vi "generate_CSV.vi"(11 "Array":string[](array[string])) -> (4 "error out":errorcluster)   [LabVIEW 2020, in "FBN_LATM.lvlib"]
uses:
  FBN_LATM.lvlib
  <vilib>/Utility/file.llb/Write Delimited Spreadsheet (string).vi
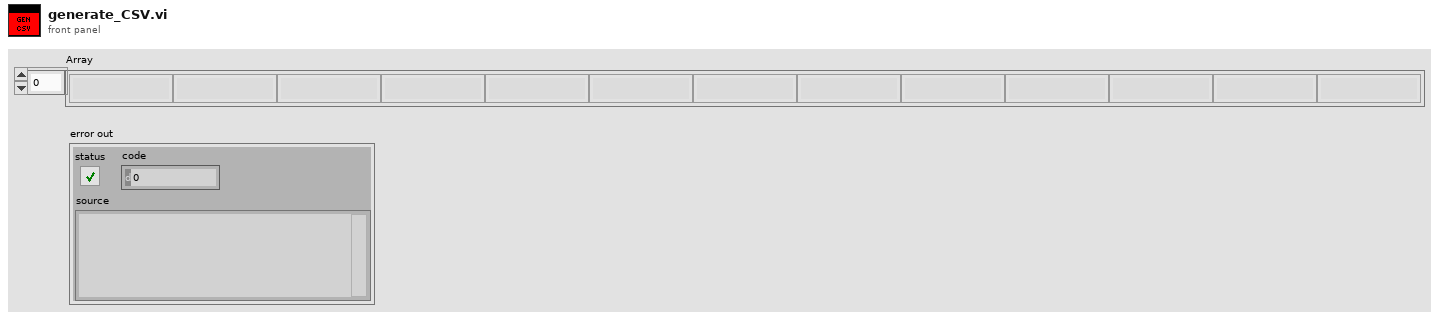
[diagram p1: front panel]
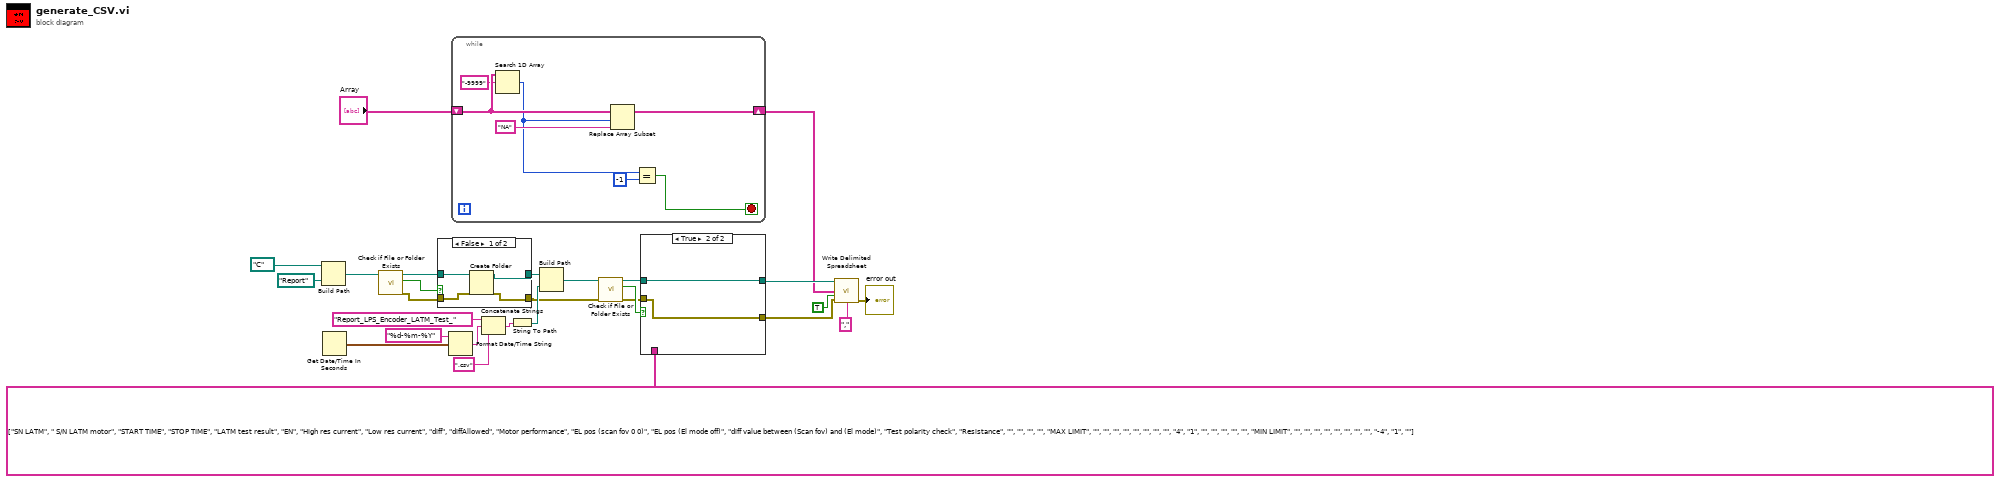
[diagram p0: block diagram]
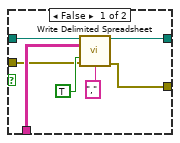
[diagram p2: hidden frame]
diagram:
  n1 = Build Path(base path=path "C:/", name or relative path=path "Report") -> (appended path=w26:path)
  n2 = Get Date/Time In Seconds() -> (seconds since 1Jan1904=w21:timestamp)
  n3 = call <vilib>:"Check if File or Folder Exists.vi"("path"=w26) -> ("error out"=w5:errorcluster, "file or folder exists?"=w24:bool, "dup path"=w25:path)  [unwired: 8 in]
  n4 = case shown="False" w24 {
    tunnel: w25 -> [w31 w33]
    tunnel: [w30 w33] -> w18
    tunnel: w5 -> [w29 w32]
    tunnel: [w28 w32] -> w4
    frame False {
      n5 = Create Folder(path (use dialog)=w31, error in=w29) -> (created path=w30:path, error out=w28:errorcluster)  [unwired: 1 in, 1 out]
    }
    frame True {
    }
  }
  n6 = Format Date/Time String(time format string (%c)="%d-%m-%Y", seconds (now)=w21) -> (date/time string=w19:string)  [unwired: 1 in]
  n7 = while {
    shift-right: [w34] -> w6
    shift-left: "Array" -> [w40]
    stop <- w35 stop-if-true
    n8 = Search 1D Array(1D array=w40, element="-9999") -> (index of element=w37:i32)  [unwired: 1 in]
    n9 = Replace Array Subset(array=w40, new element="NA" ("new element/subarray"), index=w37) -> (w34:string[])
    n10 = Equal?(x=w37, y=-1) -> (x = y?=w35:bool)
  }
  n11 = Concatenate Strings("Report_LPS_Encoder_LATM_Test_", w19, ".csv" ("string")) -> (w22:string)
  n12 = String To Path(string=w22) -> (path=w17:path)
  n13 = Build Path(base path=w18, name or relative path=w17) -> (appended path=w16:path)
  n14 = call <vilib>:"Check if File or Folder Exists.vi"("error in (no error)"=w4, "path"=w16) -> ("error out"=w3:errorcluster, "file or folder exists?"=w15:bool, "dup path"=w14:path)  [unwired: 7 in]
  n15 = case shown="True" w15 {
    tunnel: w14 -> [w45 w49]
    tunnel: [w44 w49] -> w11
    tunnel: string[][] [["SN LATM", " S/N LATM motor", "START TIME", "STOP TIME", "LATM test result", "EN", "High res current", "Low res current", "diff", "diffAllowed", "Motor performance", "EL pos (scan fov 0 0)", "EL pos (El mode off)", "diff value between (Scan fov) and (El mode)", "Test polarity check", "Resistance"], ["", "", "", "", "MAX LIMIT", "", "", "", "", "", "", "", "", "4", "1", ""], ["", "", "", "", "MIN LIMIT", "", "", "", "", "", "", "", "", "-4", "1", ""]] ("2D data") -> [w43 _]
    tunnel: w3 -> [w42 w48]
    tunnel: [w41 w48] -> w2
    frame False {
      n16 = call-poly <vilib>:"Write Delimited Spreadsheet.vi"("file path (dialog if empty)"=w45, "2D data"=w43, "append to file? (new file:F)"=TRUE, "error in (no error)"=w42, "delimiter (\\t)"="," ("delimiter (\\t)")) -> ("new file path (Not A Path if cancelled)"=w44:path, "error out"=w41:errorcluster)  [unwired: 9 in]
    }
    frame True {
    }
  }
  n17 = call-poly <vilib>:"Write Delimited Spreadsheet.vi"("file path (dialog if empty)"=w11, "1D data"=w6, "append to file? (new file:F)"=TRUE, "error in (no error)"=w2, "delimiter (\\t)"="," ("delimiter (\\t)")) -> ("error out"=→"error out":errorcluster)  [unwired: 9 in, 1 out]
